vi "DataCut(Ver.3).vi"(1 "Input data array":dbl[](array[numeric])) -> (0 "Output data array":dbl[](array[numeric]))   [LabVIEW 2016]
panel:
  out "反転配列":dbl[](array[numeric])
  out "number of data":i32
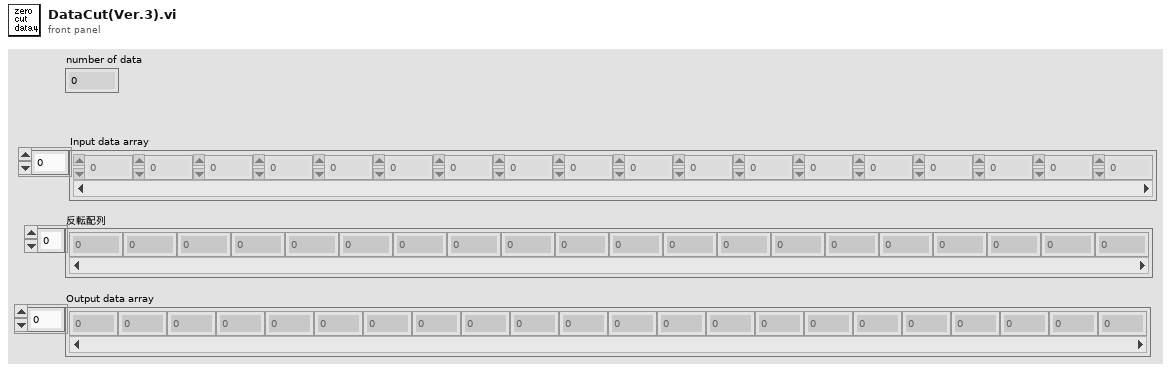
[diagram p1: front panel]
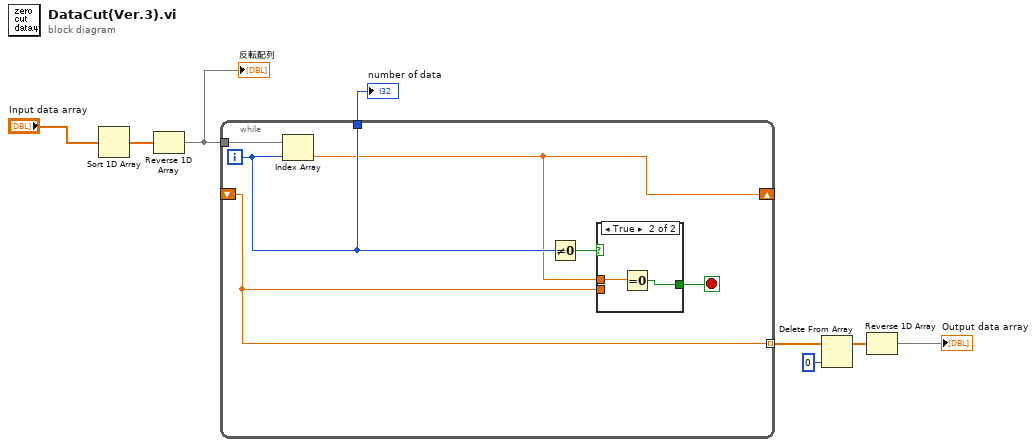
[diagram p0: block diagram]
diagram:
  n1 = Sort 1D Array(array="Input data array") -> (sorted array=w6:dbl[])
  n2 = Reverse 1D Array(array=w6) -> (reversed array=w5:dbl[])
  "反転配列" <- w5
  n3 = while {
    shift-right: [w10] -> _
    shift-left: _ -> [w9]
    tunnel: w5 -> [w13]
    tunnel: [w11] -> w8
    tunnel: [w9] -> w3 mode=indexing
    i -> [w11]
    stop <- w14 stop-if-true
    n4 = Index Array(array=w13, index=w11) -> (element=w10:dbl)
    n5 = Not Equal To 0?(x=w11) -> (x != 0?=w12:bool)
    n6 = case shown="True" w12 {
      tunnel: [_ w15] -> w14
      tunnel: w9 -> [_ _]
      tunnel: w10 -> [_ w16]
      frame False {
      }
      frame True {
        n7 = Equal To 0?(x=w16) -> (x = 0?=w15:bool)
      }
    }
  }
  "number of data" <- w8
  n8 = Delete From Array(array=w3, index=0) -> (array with subset deleted=w1:dbl[])  [unwired: 1 in, 1 out]
  n9 = Reverse 1D Array(array=w1) -> (reversed array=→"Output data array":dbl[])
